vi "New.vi"(8 "error in (no error)":errorcluster, 10 "Parent":refnum<class "Config Element.lvclass">, 11 "Name":string) -> (0 "error out":errorcluster, 3 "Cluster out":refnum<class "Cluster.lvclass">)   [LabVIEW 2020, in "VolatusConfig.lvlib" / "Cluster.lvclass"]
uses:
  Cluster.lvclass
  lv-cdm/CDM-Config/Config Element/Config Element.lvclass
  lv-cdm/CDM-Config/Value Type.ctl
  lv-cdm/CDM-Config/CDM-Config.lvlib
  VolatusConfigElement/VolatusConfigElement.lvclass
  VolatusConfig.lvlib
  Meta Type.ctl
  C:/dev/lv20CE/relink/lv-volatus/VolatusConfig/VolatusConfigElement/VolatusConfigElement.lvclass
  C:/dev/lv20CE/relink/lv-volatus/VolatusConfig/Cluster/Cluster.lvclass
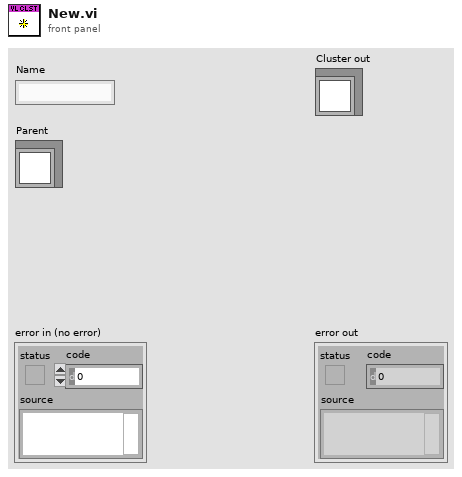
[diagram p1: front panel]
types:
  T1 = typedef "CDM-Config.lvlib/Value Type.ctl" = enum16{"String", "Number", "Bool", "Object", "Array"}
  T2 = typedef "VolatusConfig.lvlib/Meta Type.ctl" = enum16{"UNKNOWN", "VL_System", "VL_Cluster", "VL_Node", "VL_Task", "VL_Group", "VL_Channel", "VL_Task_List", "VL_Scaling", "VL_Sensor", "VL_Sensor_List", "VL_Scale"}
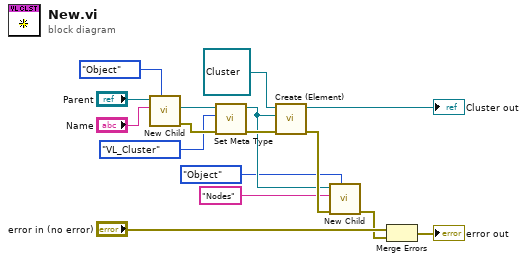
[diagram p0: block diagram]
diagram:
  n1 = call "New Child.vi"("Value Type (String)"=Value_Type."Object", "Child Name"="Name", "Config Element in"="Parent") -> ("error out"=w15:errorcluster, "New Child"=w10:refnum<class "Config Element.lvclass">)  [unwired: 6 in, 1 out]
  n2 = call "Set Meta Type.vi"("error in (no error)"=w15, "Meta Type"=Meta_Type."VL_Cluster", "Element In"=w10) -> ("error out"=w8:errorcluster, "Element"=w4:refnum<class "Config Element.lvclass">)  [unwired: 7 in]
  n3 = call "Create (Element).vi"("error in (no error)"=w8, "Element"=w4, "VolatusConfigElement in"=refnum<class "Cluster.lvclass"> refnum ("Cluster in")) -> ("error out"=w16:errorcluster, "VolatusConfigElement out"=→"Cluster out":refnum<class "Cluster.lvclass">)  [unwired: 7 in]
  n4 = call "New Child.vi"("Value Type (String)"=Value_Type."Object", "error in (no error)"=w16, "Child Name"="Nodes", "Config Element in"=w4) -> ("error out"=w1:errorcluster)  [unwired: 5 in, 2 out]
  n5 = Merge Errors("error in (no error)", w1) -> (→"error out":errorcluster)
